vi "Set step.vi"(8 "error in (no error)":errorcluster, 9 "Step":dbl=2.0, 10 "Address":dbl=1.0, 11 "VISA resource name (IN)":refnum<visa-resource-name>) -> (0 "error out":errorcluster, 3 "VISA resource name (OUT)":refnum<visa-resource-name>)   [LabVIEW 2010, in "Yudian AI508.lvlib"]
doc: "Use this template to build a VI to use as a subVI."
uses:
  <instrlib>/Yudian AI508/Yudian AI508.lvlib
panel:
  out "Recieved Raw Data":string
  out "Recevied Temp.  data":dbl
  out "Data buffer":string
  out "Digital shift":i32
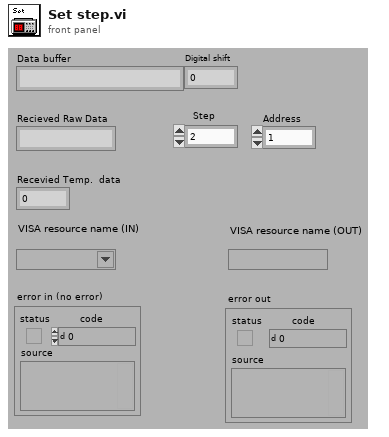
[diagram p1: front panel]
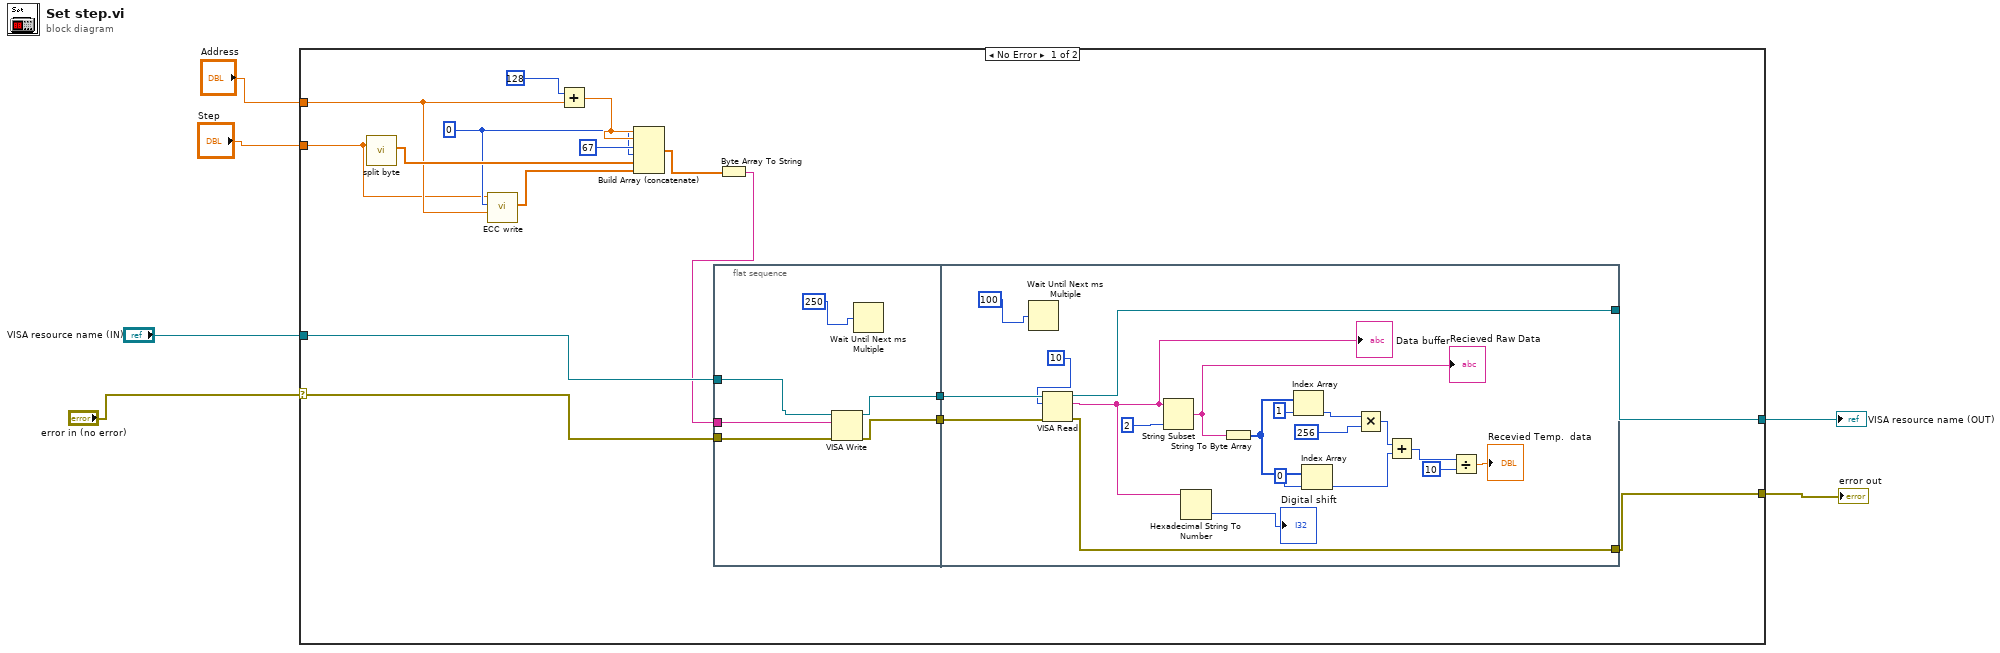
[diagram p0: block diagram]
diagram:
  n1 = case shown="No Error" "error in (no error)" {
    selector: "error in (no error)" -> [w17 w50]
    tunnel: [w19 w50] -> w6
    tunnel: [w20 w49] -> w5
    tunnel: "VISA resource name (IN)" -> [w18 w49]
    tunnel: "Step" -> [w8 _]
    tunnel: "Address" -> [w9 _]
    frame No Error {
      w11 = 0
      n2 = call <instrlib>:"split byte.vi"("Value"=w8) -> ("Array"=w12:dbl[])  [unwired: 10 in]
      n3 = call <instrlib>:"ECC write.vi"("Address"=w9, "Parameter code"=w11, "Value"=w8) -> ("Data array"=w10:dbl[])  [unwired: 8 in]
      n4 = Add(x=128, y=w9) -> (x+y=w15:dbl)
      n5 = Build Array (concatenate)(w15, w15, 67, w11, w12, w10) -> (w7:dbl[])
      n6 = flat-sequence {
        tunnel: w17 -> [w28]
        tunnel: w18 -> [w25]
        tunnel: [w27] -> w22
        tunnel: [w26] -> w21
        tunnel: w16 -> [w23]
        tunnel: w22 -> [w34]
        tunnel: w21 -> [w33]
        tunnel: [w31] -> w20
        tunnel: [w30] -> w19
        frame #0 {
          n7 = VISA Write(VISA resource name=w25, write buffer=w23, error in (no error)=w28) -> (VISA resource name out=w26:refnum<visa-resource-name>, error out=w27:errorcluster)  [unwired: 1 out]
          n8 = Wait Until Next ms Multiple(millisecond multiple=250) -> ()  [unwired: 1 out]
        }
        frame #1 {
          n9 = Wait Until Next ms Multiple(millisecond multiple=100) -> ()  [unwired: 1 out]
          n10 = VISA Read(VISA resource name=w33, byte count=u32 10 ("字节总数"), error in (no error)=w34) -> (VISA resource name out=w31:refnum<visa-resource-name>, read buffer=w36:string, error out=w30:errorcluster)  [unwired: 1 out]
          "Data buffer" <- w36
          n11 = String Subset(string=w36, length (rest)=2 ("length (rest)")) -> (substring=w46:string)  [unwired: 1 out]
          "Recieved Raw Data" <- w46
          n12 = Hexadecimal String To Number(string=w36) -> (number=→"Digital shift":u32)  [unwired: 3 out]
          n13 = String To Byte Array(string=w46) -> (unsigned byte array=w44:u8[])
          n14 = Index Array(array=w44, index=1) -> (element=w43:u8)
          n15 = Index Array(array=w44, index=0) -> (element=w40:u8)
          n16 = Multiply(x=w43, y=u16 256) -> (x*y=w41:u16)
          n17 = Add(x=w41, y=w40) -> (x+y=w39:u16)
          n18 = Divide(x=w39, y=u16 10) -> (x/y=→"Recevied Temp.  data":dbl)
        }
      }
      n19 = Byte Array To String(unsigned byte array=w7) -> (string=w16:string)
    }
    frame Error {
    }
  }
  "error out" <- w6
  "VISA resource name (OUT)" <- w5
